vi "Do.vi"(8 "error in (no error)":errorcluster, 10 "Actor in":refnum<class "Actor.lvclass">, 11 "New Results Msg":refnum<class "New Results Msg.lvclass">) -> (0 "error out":errorcluster, 2 "Actor out":refnum<class "Actor.lvclass">)   [LabVIEW 2014, in "HIJ Vision Display.lvlib" / "New Results Msg.lvclass"]
doc: "This VI delivers the message to the actor by calling the appropriate method(s) on the actor."
uses:
  New Results Msg.lvclass
  <vilib>/ActorFramework/Actor/Actor.lvclass
  HIJ Vision Display/HIJ Vision Display.lvclass
  Abstract Messages/Publish Analyze Results Msg/Publish Analyze Results Msg.lvclass/Publish Analyze Results Msg.ctl
  Abstract Messages/Publish Analyze Results Msg/Publish Analyze Results Msg.lvclass
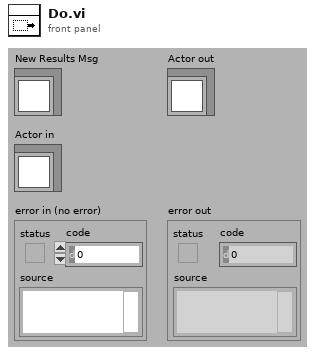
[diagram p1: front panel]
types:
  T1 = cluster{"Image Nr.":i32, "Results":refnum<class "Analyze Results Base.lvclass">[], "Parameters":refnum<class "Analyze Parameter Base.lvclass">[]}
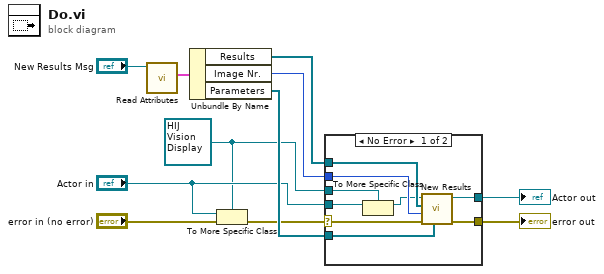
[diagram p0: block diagram]
diagram:
  w5 = refnum<class "HIJ Vision Display.lvclass"> refnum ("Actor in")
  n1 = call "Read Attributes.vi"("Abstract Message Template in"="New Results Msg") -> ("Payload"=w3:T1)  [unwired: 9 in, 1 out]
  n2 = Unbundle By Name(w3) -> ("Results"=w2:refnum<class "Analyze Results Base.lvclass">[], "Image Nr."=w1:i32, "Parameters"=w11:refnum<class "Analyze Parameter Base.lvclass">[])
  n3 = To More Specific Class(target class=w5, reference="Actor in", error in="error in (no error)") -> (error out=w9:errorcluster)  [unwired: 1 out]
  n4 = case shown="No Error" w9 {
    selector: w9 -> [w18 w22]
    tunnel: [w20 w22] -> w8
    tunnel: [w19 w21] -> w7
    tunnel: "Actor in" -> [w17 w21]
    tunnel: w5 -> [w16 _]
    tunnel: w2 -> [w15 _]
    tunnel: w1 -> [w14 _]
    tunnel: w11 -> [w12 _]
    frame No Error {
      n5 = To More Specific Class(target class=w16, reference=w17) -> (specific class reference=w13:refnum<class "HIJ Vision Display.lvclass">)  [unwired: 1 in, 1 out]
      n6 = call-dynamic "New Results.vi"("Parameters"=w12, "error in (no error)"=w18, "Image Nr."=w14, "Results"=w15, "HIJ Vision Display in"=w13) -> ("error out"=w20:errorcluster, "HIJ Vision Display out"=w19:refnum<class "HIJ Vision Display.lvclass">)  [unwired: 5 in]
    }
    frame Error {
    }
  }
  "error out" <- w8
  "Actor out" <- w7
